vi "Get_computername.vi"(8 "error in (no error)":errorcluster) -> (0 "error out":errorcluster, 2 "Computer Name":string)   [LabVIEW 2018]
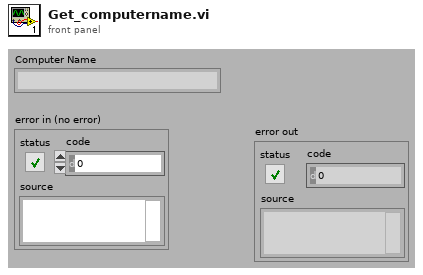
[diagram p1: front panel]
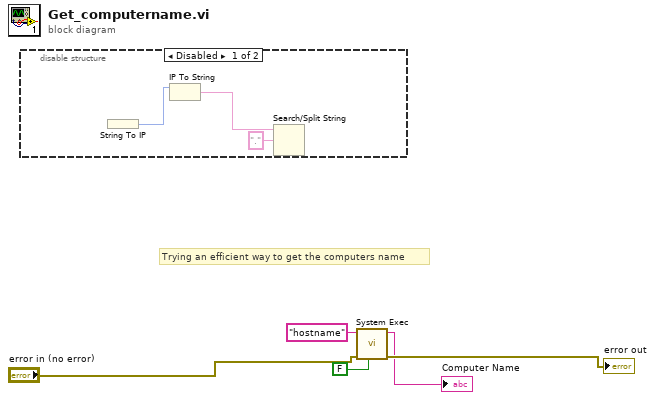
[diagram p0: block diagram]
diagram:
  # "Trying an efficient way to get the computers name"
  n1 = disable-structure shown="Disabled" {
    frame Disabled {
      n2 = String To IP() -> (0:w7:u32)  [unwired: 1 in]
      n3 = IP To String(2:w7) -> (0:w6:string)  [unwired: 1 in]
      n4 = Search/Split String(string=w6, search string/char (-)=".") -> ()  [unwired: 1 in, 3 out]
    }
    frame Enabled {
    }
  }
  n5 = call <vilib>:"System Exec.vi"("run minimized? (F)"=FALSE, "error in (no error)"="error in (no error)", "command line"="hostname") -> ("error out"=→"error out":errorcluster, "standard output"=→"Computer Name":string)  [unwired: 5 in, 2 out]
